vi "Set Default SplitViPath.vi"(8 "error in (no error)":errorcluster caption="错误输入（无错误）", 11 "PanelDataNode 输入":refnum<class "PanelDataNode.lvclass"> caption="DNL_LabVIEW Object in") -> (0 "error out":errorcluster caption="错误输出", 3 "PanelDataNode 输出":refnum<class "PanelDataNode.lvclass"> caption="DNL_LabVIEW Object out")   [LabVIEW 2013, in "PanelDataNode.lvclass"]
uses:
  PanelDataNode.lvclass
  PanelDataNode.lvclass/PanelDataNode.ctl
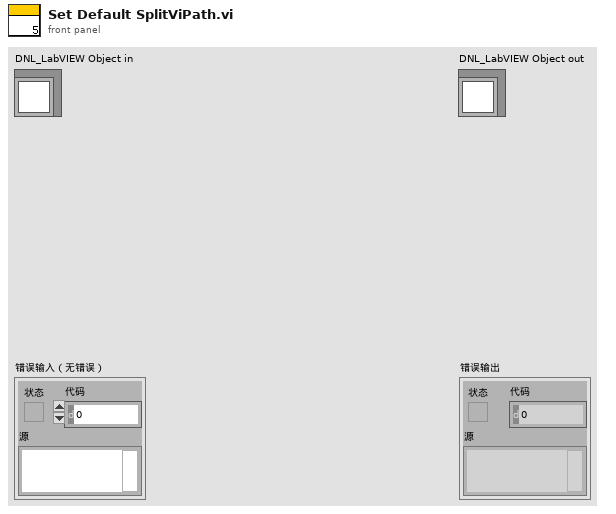
[diagram p1: front panel]
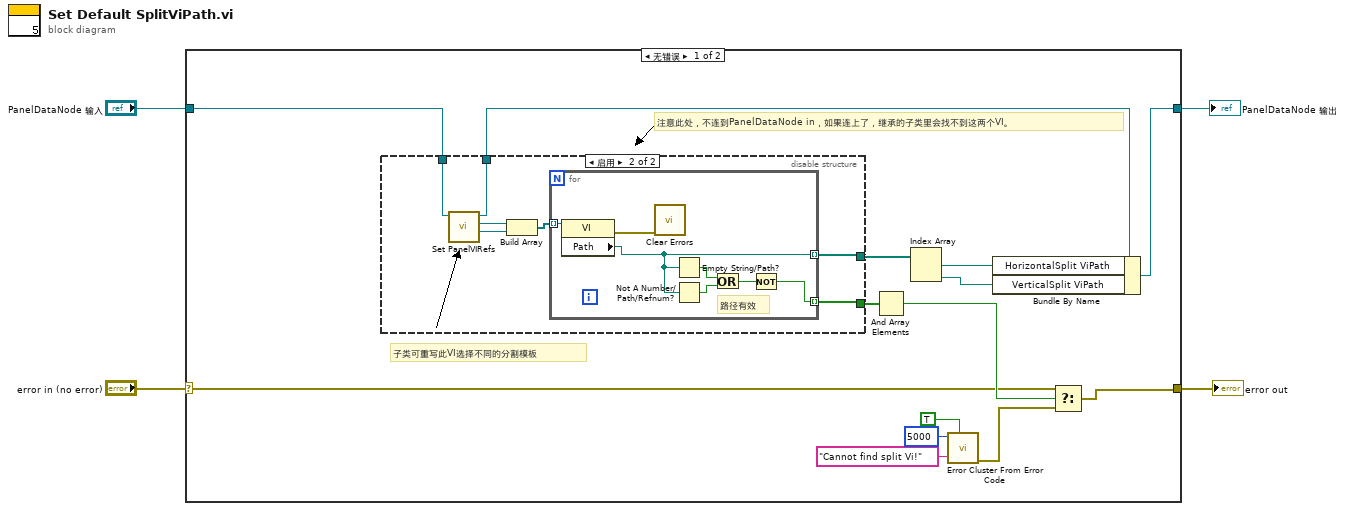
[diagram p0: block diagram]
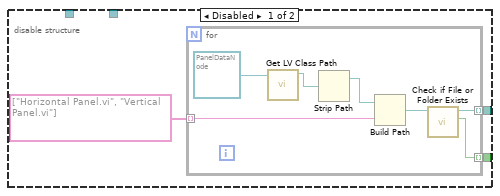
[diagram p2: hidden frame]
diagram:
  n1 = case shown="无错误" "error in (no error)" {
    selector: "error in (no error)" -> [w12 w44]
    tunnel: [w11 w44] -> w3
    tunnel: [w15 w43] -> w1
    tunnel: "PanelDataNode 输入" -> [w6 w43]
    frame No Error {
      # "子类可重写此VI选择不同的分割模板"
      # "注意此处，不连到PanelDataNode in，如果连上了，继承的子类里会找不到这两个VI。"
      n2 = disable-structure shown="启用" {
        disable-tunnel: [w21 w35] -> w18
        disable-tunnel: [w19 w34] -> w14
        disable-tunnel: w6 -> [_ w33]
        disable-tunnel: [_ w32] -> w5
        frame Disabled {
          n3 = for {
            tunnel: [w24] -> w21 mode=indexing
            tunnel: string[] ["Horizontal Panel.vi", "Vertical Panel.vi"] -> [w26] mode=indexing
            tunnel: [w23] -> w19 mode=indexing
            n4 = call <vilib>:"Get LV Class Path.vi"("object"=refnum<class "PanelDataNode.lvclass"> refnum ("PanelDataNode.lvclass")) -> ("class path"=w27:path)  [unwired: 9 in, 1 out]
            n5 = Strip Path(path=w27) -> (stripped path=w28:path)  [unwired: 1 out]
            n6 = Build Path(base path=w28, name or relative path=w26) -> (appended path=w25:path)
            n7 = call <vilib>:"Check if File or Folder Exists.vi"("path"=w25) -> ("file or folder exists?"=w23:bool, "dup path"=w24:path)  [unwired: 8 in, 1 out]
          }
        }
        frame Enabled {
          n8 = call-dynamic "Set PanelVIRefs.vi"("PanelDataNode 输入"=w33) -> ("VerticalPanel"=w29:refnum<vi>, "HorizontalPanel"=w30:refnum<vi>, "PanelDataNode 输出"=w32:refnum<class "PanelDataNode.lvclass">)  [unwired: 7 in, 1 out]
          n9 = Build Array(w30, w29) -> (w31:refnum<vi>[])
          n10 = for {
            tunnel: [w41] -> w35 mode=indexing
            tunnel: [w37] -> w34 mode=indexing
            tunnel: w31 -> [w42] mode=indexing
            # "路径有效"
            n11 = property class="VI"(reference=w42) -> (error out=w36:errorcluster, "Path"=w41:path)  [unwired: 1 in, 1 out]
            n12 = call <vilib>:"Clear Errors.vi"("error in (no error)"=w36) -> ()  [unwired: 6 in, 1 out]
            n13 = Empty String/Path?(string/path=w41) -> (empty?=w39:bool)
            n14 = Not A Number/Path/Refnum?(number/path/refnum=w41) -> (NaN/Path/Refnum?=w40:bool)
            n15 = Or(x=w39, y=w40) -> (x .or. y?=w38:bool)
            n16 = Not(x=w38) -> (.not. x?=w37:bool)
          }
        }
      }
      n17 = And Array Elements(Boolean array=w14) -> (logical AND=w13:bool)
      n18 = Index Array(array=w18) -> (element #1=w17:path, element #2=w16:path)  [unwired: 2 in]
      n19 = call <vilib>:"Error Cluster From Error Code.vi"("show call chain? (False)"=TRUE, "error message (\"\")"="Cannot find split Vi!" ("error message (\"\")"), "error code (0)"=5000) -> ("error out"=w8:errorcluster)  [unwired: 6 in]
      n20 = Bundle By Name(cluster=w5, "HorizontalSplit ViPath"=w17, "VerticalSplit ViPath"=w16) -> (w15:refnum<class "PanelDataNode.lvclass">)
      n21 = Select(t=w12, s=w13, f=w8) -> (s? t:f=w11:errorcluster)
    }
    frame Error {
    }
  }
  "error out" <- w3
  "PanelDataNode 输出" <- w1
